vi "Output on.vi"(8 "error in (no error)":errorcluster, 10 "Output On":bool, 11 "Manual PSU in":refnum<class "Manual PSU.lvclass">) -> (0 "error out":errorcluster, 3 "Manual PSU out":refnum<class "Manual PSU.lvclass">)   [LabVIEW 2020, in "Manual PSU.lvclass"]
uses:
  Manual PSU.lvclass
  C:/Sandbox/Git_Sandbox/WiSpry Test Framework source code (LV20)/WiSpry Test Framework/Instruments/Power Supply/Power Supply.lvclass
  Power Supply.lvclass/Power Supply.ctl
  Power Supply.lvclass
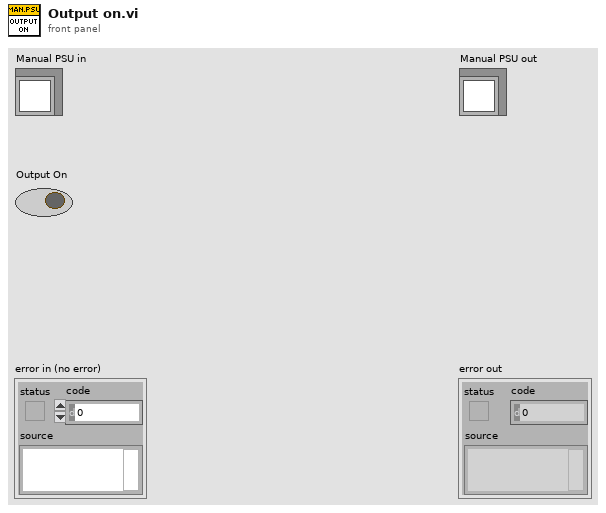
[diagram p1: front panel]
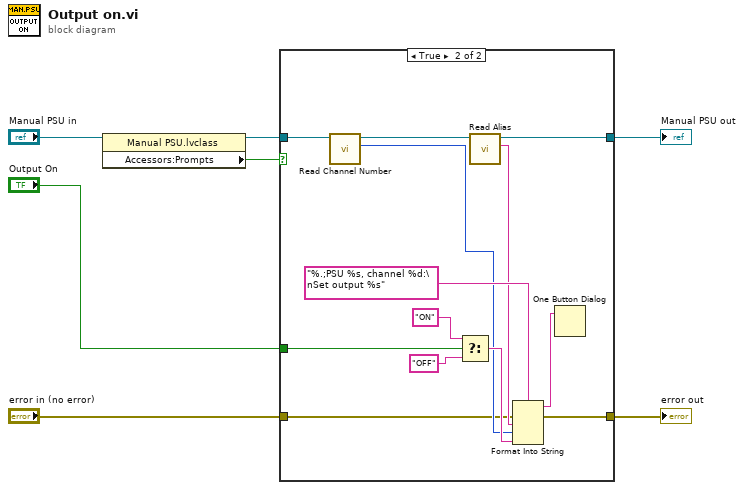
[diagram p0: block diagram]
diagram:
  n1 = property class="Manual PSU.lvclass"(reference="Manual PSU in") -> (reference out=w2:refnum<class "Manual PSU.lvclass">, "Accessors:Prompts"=w1:bool)  [unwired: 1 in, 1 out]
  n2 = case shown="True" w1 {
    tunnel: "error in (no error)" -> [w9 w16]
    tunnel: [w9 w15] -> w6
    tunnel: [w8 w14] -> w5
    tunnel: "Output On" -> [_ w13]
    tunnel: w2 -> [w8 w10]
    frame False {
    }
    frame True {
      n3 = call "Read Channel Number.vi"("Power Supply in"=w10) -> ("Channel Number"=w17:u8, "Power Supply out"=w18:refnum<class "Manual PSU.lvclass">)  [unwired: 9 in]
      n4 = Select(t="ON" ("format string"), s=w13, f="OFF" ("format string")) -> (s? t:f=w20:string)
      n5 = call-dynamic "Read Alias.vi"("Power Supply in"=w18) -> ("Alias"=w19:string, "Power Supply out"=w14:refnum<class "Manual PSU.lvclass">)  [unwired: 9 in]
      n6 = Format Into String(format string="%.;PSU %s, channel %d:\nSet output %s", error in=w16, w19, w17, w20) -> (resulting string=w21:string, error out=w15:errorcluster)  [unwired: 1 in]
      n7 = One Button Dialog(message=w21) -> ()  [unwired: 1 in, 1 out]
    }
  }
  "error out" <- w6
  "Manual PSU out" <- w5
